vi "Move Reference.vi"(4 "Side":T1=enum."right", 5 "Label":string, 6 "Wait Time":dbl, 8 "error in":errorcluster, 9 "Time":dbl, 10 "To Reference":bool=TRUE, 11 "Object":string) -> (0 "error out":errorcluster)   [LabVIEW 2013]
uses:
  ROS/Code/SubVIs/BaxterSide.ctl
  Arm Globals.vi
  ROS/Code/Console/Servers/ServerSubs/(nist) Arm Globals.vi
panel:
  in  "ByPass":bool=TRUE
  # "Dummy Input\nto mark\npolymorphic\noption"
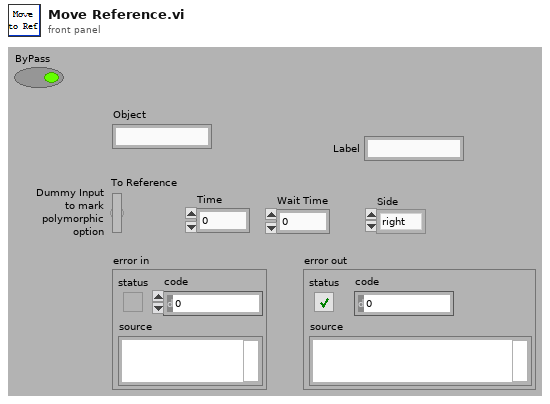
[diagram p1: front panel]
types:
  T1 = typedef "BaxterSide.ctl" = enum16{"left", "right"}
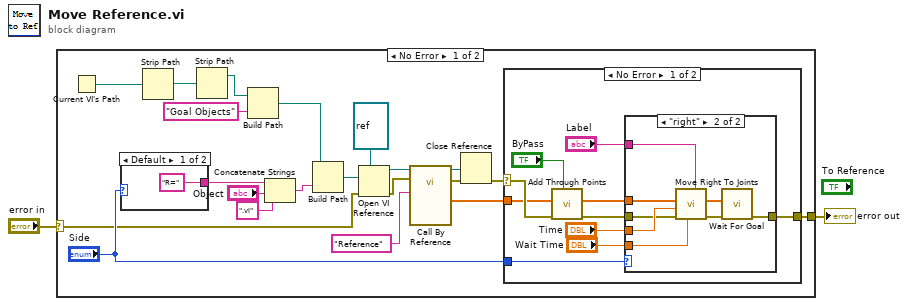
[diagram p0: block diagram]
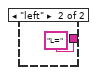
[diagram p2: hidden frame]
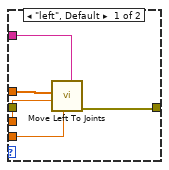
[diagram p3: hidden frame]
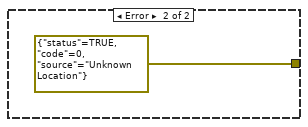
[diagram p4: hidden frame]
diagram:
  n1 = case shown="No Error" "error in" {
    selector: "error in" -> [w3 w50]
    tunnel: [w23 w50] -> w1
    frame No Error {
      n2 = Current VI's Path() -> (path=w8:path)
      n3 = case shown="Default" "Side" {
        tunnel: ["R=" "L="] -> w20
        frame Default {
        }
        frame "left" {
        }
      }
      n4 = Strip Path(path=w8) -> (stripped path=w7:path)  [unwired: 1 out]
      n5 = Strip Path(path=w7) -> (stripped path=w6:path)  [unwired: 1 out]
      n6 = Build Path(base path=w6, name or relative path="Goal Objects") -> (appended path=w4:path)
      n7 = Concatenate Strings(w20, "Object", ".vi" ("string")) -> (w10:string)
      n8 = Build Path(base path=w4, name or relative path=w10) -> (appended path=w9:path)
      n9 = Open VI Reference(type specifier VI Refnum (for type only)=refnum<vi> refnum, vi path=w9, error in (no error)=w3) -> (vi reference=w17:refnum<vi>, error out=w14:errorcluster)  [unwired: 3 in]
      n10 = call-by-ref "?"(reference=w17, error in=w14, "Command"="Reference") -> (reference out=w15:refnum<vi>, error out=w13:errorcluster, "Joints"=w11:dbl[])  [unwired: 8 in, 2 out]
      n11 = Close Reference(reference=w15, error in (no error)=w13) -> (error out=w12:errorcluster)
      n12 = case shown="No Error" w12 {
        selector: w12 -> [w29 _]
        tunnel: [w33 errorcluster {"status"=TRUE, "code"=0, "source"="Unknown Location"} ("error out")] -> w23
        tunnel: "Side" -> [w31 _]
        tunnel: w11 -> [w28 _]
        frame No Error {
          n13 = call "Add Through Points.vi"("ByPass"="ByPass", "error in"=w29, "Goal"=w28) -> ("error out"=w30:errorcluster, "Goal"=w27:dbl[])  [unwired: 7 in]
          n14 = case shown="\"right\"" w31 {
            tunnel: "Time" -> [w37 w45]
            tunnel: "Label" -> [w39 w47]
            tunnel: [w40 w41] -> w33
            tunnel: w27 -> [w38 w46]
            tunnel: "Wait Time" -> [w36 w48]
            tunnel: w30 -> [_ w44]
            frame "left", Default {
              n15 = call "Move Left To Joints.vi"("Label"=w39, "Wait (s)"=w36, "time"=w37, "Goal"=w38) -> ("error out"=w40:errorcluster)  [unwired: 6 in, 1 out]
            }
            frame "right" {
              n16 = call "Move Right To Joints.vi"("Label"=w47, "Wait (s)"=w48, "error in"=w44, "time"=w45, "Goal"=w46) -> ("error out"=w43:errorcluster, "Goal"=w42:dbl[])  [unwired: 5 in]
              n17 = call "Wait For Goal.vi"("error in"=w43, "Goal"=w42) -> ("error out"=w41:errorcluster)  [unwired: 8 in, 1 out]
            }
          }
        }
        frame Error {
        }
      }
    }
    frame Error {
    }
  }
  "error out" <- w1
